vi "FieldOrientedTransform.vi"(7 "Orientation Mode":T1(ring), 9 "Joystick Y":dbl, 11 "Joystick X":dbl) -> (1 "Joystick Y'":dbl, 3 "Joystick X'":dbl)   [LabVIEW 2020]
doc: "Transforms X and Y joystick axes based on the robot's current orientation, allowing a swerve robot to be controlled in the field-oriented reference frame. The code is primarily based on code included in the FRC WPI Library."
uses:
  sensordata.vi
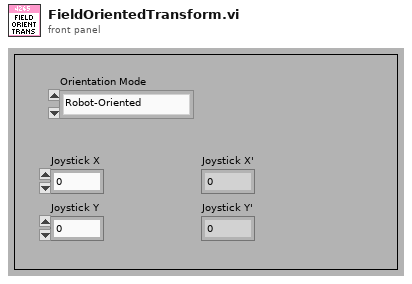
[diagram p1: front panel]
types:
  T1 = enum16{"Robot-Oriented", "Field-Oriented", "Intake"}
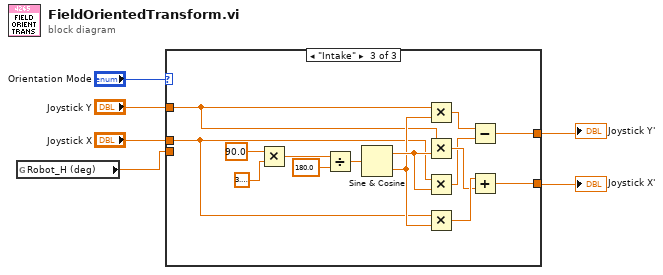
[diagram p0: block diagram]
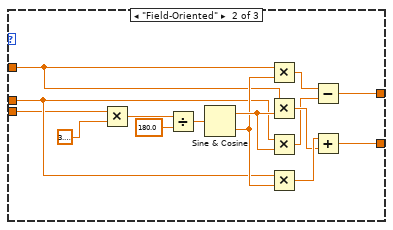
[diagram p3: hidden frame]
diagram:
  n1 = global read "sensordata.vi" "Robot_H (deg)"() -> (w2:dbl)
  n2 = case shown="\"Intake\"" "Orientation Mode" {
    tunnel: "Joystick Y" -> [w8 w15 w30]
    tunnel: "Joystick X" -> [w7 w14 w29]
    tunnel: w2 -> [_ w12 _]
    tunnel: [w8 w11 w27] -> w4
    tunnel: [w7 w10 w26] -> w3
    frame "Robot-Oriented", Default {
      # "robot-oriented"
    }
    frame "Field-Oriented" {
      # "field-oriented"
      n3 = Multiply(x=w12, y=3.141592653589793) -> (x*y=w23:dbl)
      n4 = Divide(x=w23, y=180.0) -> (x/y=w22:dbl)
      n5 = Sine & Cosine(0:w22) -> (1:w19:dbl, 2:w18:dbl)
      n6 = Multiply(x=w15, y=w18) -> (x*y=w17:dbl)
      n7 = Multiply(x=w15, y=w19) -> (x*y=w20:dbl)
      n8 = Multiply(x=w14, y=w19) -> (x*y=w16:dbl)
      n9 = Multiply(x=w14, y=w18) -> (x*y=w21:dbl)
      n10 = Subtract(x=w17, y=w16) -> (x-y=w11:dbl)
      n11 = Add(x=w21, y=w20) -> (x+y=w10:dbl)
    }
    frame "Intake" {
      # "field-oriented"
      n12 = Multiply(x=90.0, y=3.141592653589793) -> (x*y=w38:dbl)
      n13 = Divide(x=w38, y=180.0) -> (x/y=w37:dbl)
      n14 = Sine & Cosine(0:w37) -> (1:w34:dbl, 2:w33:dbl)
      n15 = Multiply(x=w30, y=w33) -> (x*y=w32:dbl)
      n16 = Multiply(x=w30, y=w34) -> (x*y=w35:dbl)
      n17 = Multiply(x=w29, y=w34) -> (x*y=w31:dbl)
      n18 = Multiply(x=w29, y=w33) -> (x*y=w36:dbl)
      n19 = Subtract(x=w32, y=w31) -> (x-y=w27:dbl)
      n20 = Add(x=w36, y=w35) -> (x+y=w26:dbl)
    }
  }
  "Joystick Y'" <- w4
  "Joystick X'" <- w3
